vi "3.vi"() -> ()   [LabVIEW 2019]
uses:
  <vilib>/imath/engines/lvmath/Plug In/_Char/NIMS_CH_character datatype.ctl
  <vilib>/imath/engines/lvmath/Plug In/_Char/NIMS_CH_Character RV to String.vi
  <vilib>/imath/engines/lvmath2/RunTimeEngine/BuiltInFunctions/random/NIMS_random.vi
  <vilib>/imathl/engines/lvmath/Functions/Error Handling/Create Error.vi
  <vilib>/imath/engines/lvmath2/RunTimeEngine/BuiltInFunctions/fir_win/NIMS_fir_win(I32,V,Str,V,Str).vi
  <vilib>/imath/engines/lvmath2/RunTimeEngine/ErrorHandling/NIMS_Create Error From Enums.vi
  <vilib>/imath/engines/lvmath2/RunTimeEngine/BuiltInFunctions/fft/NIMS_fft(GV).vi
  <instcachedir>/0/NIMS_fft(GV)_4C6467FC22F84E4BA42517A07EF978B0.lvgen/NIMS_fft(GV)_4C6467FC22F84E4BA42517A07EF978B0_000.vi
  <vilib>/imath/engines/lvmath2/RunTimeEngine/ErrorHandling/NIMS_Error From Error Code.vi
  <vilib>/imath/engines/lvmath2/RunTimeEngine/RangeToken/NIMS_Range.vi
  <instcachedir>/0/NIMS_Range_FADF6ADDA3E145BB934C8BD4C7DAAB97.lvgen/NIMS_Range_FADF6ADDA3E145BB934C8BD4C7DAAB97_000.vi
  <vilib>/imath/engines/lvmath2/RunTimeSupport/NIMS_Error if Not Equal.vi
  <instcachedir>/0/NIMS_Error if Not Equal_D50A0F08CBFC40E0B64682CCD852CBC7.lvgen/NIMS_Error if Not Equal_D50A0F08CBFC40E0B64682CCD852CBC7_001.vi
  <vilib>/imath/engines/lvmath2/RunTimeEngine/IndexRead/NIMS V(V).vi
  <instcachedir>/0/NIMS V(V)_298D9CB7BFEB42B8BC8D9C3C28AE8C70.lvgen/NIMS V(V)_298D9CB7BFEB42B8BC8D9C3C28AE8C70_001.vi
  <vilib>/imath/engines/lvmath2/RunTimeEngine/BuiltInFunctions/abs/NIMS_abs(signed).vi
  <instcachedir>/0/NIMS_abs(signed)_C4FCB8E6058B49B797C7C8D53CA5F6EC.lvgen/NIMS_abs(signed)_C4FCB8E6058B49B797C7C8D53CA5F6EC_006.vi
  <vilib>/imath/engines/lvmath2/RunTimeEngine/BuiltInFunctions/crosscorr/NIMS_crosscorr(GM,Str).vi
  <instcachedir>/0/NIMS_crosscorr(GM,Str)_7E3A3CE9917B451394D0C3CD4C3D6955.lvgen/NIMS_crosscorr(GM,Str)_7E3A3CE9917B451394D0C3CD4C3D6955_000.vi
  <vilib>/imath/engines/lvmath2/RunTimeEngine/BuiltInFunctions/fft/NIMS_fft(GM).vi
  <instcachedir>/0/NIMS_fft(GM)_17D9014FFEBE444196AC5CE36A7D9342.lvgen/NIMS_fft(GM)_17D9014FFEBE444196AC5CE36A7D9342_000.vi
  <vilib>/imath/engines/lvmath2/RunTimeEngine/ArithmeticOperatorToken/NIMS_ArithmeticOperator_power(S).vi
  <instcachedir>/0/NIMS_ArithmeticOperator_power(S)_F1497A2DE3CE4E82B2C3646D59904248.lvgen/NIMS_ArithmeticOperator_power(S)_F1497A2DE3CE4E82B2C3646D59904248_012.vi
  <vilib>/imath/engines/lvmath2/RunTimeEngine/ArithmeticOperatorToken/NIMS_ArithmeticOperator_times.vi
  <instcachedir>/0/NIMS_ArithmeticOperator_times_B08792E9E3A74C8190DF4DEBB44E818C.lvgen/NIMS_ArithmeticOperator_times_B08792E9E3A74C8190DF4DEBB44E818C_007.vi
  <vilib>/imath/engines/lvmath2/RunTimeEngine/BuiltInFunctions/ifft/NIMS_ifft(CM).vi
  <vilib>/imath/engines/lvmath2/RunTimeEngine/BuiltInFunctions/fftshift/NIMS_fftshift(GM).vi
  <vilib>/imath/engines/lvmath2/RunTimeEngine/IndexRead/NIMS M(V).vi
  <instcachedir>/0/NIMS M(V)_948FAC22C1C943948B75DA6190348614.lvgen/NIMS M(V)_948FAC22C1C943948B75DA6190348614_005.vi
  <instcachedir>/0/NIMS_abs(signed)_C4FCB8E6058B49B797C7C8D53CA5F6EC.lvgen/NIMS_abs(signed)_C4FCB8E6058B49B797C7C8D53CA5F6EC_005.vi
  <instcachedir>/0/NIMS V(V)_298D9CB7BFEB42B8BC8D9C3C28AE8C70.lvgen/NIMS V(V)_298D9CB7BFEB42B8BC8D9C3C28AE8C70_000.vi
  <instcachedir>/0/NIMS_abs(signed)_C4FCB8E6058B49B797C7C8D53CA5F6EC.lvgen/NIMS_abs(signed)_C4FCB8E6058B49B797C7C8D53CA5F6EC_001.vi
  <vilib>/imath/engines/lvmath2/RunTimeEngine/NodeEndStatement/NIMS_NodeEndStatement_Get Vector.vi
  <instcachedir>/0/NIMS_NodeEndStatement_Get Vector_92F29E6578CC4FEABDAC0B727A70E862.lvgen/NIMS_NodeEndStatement_Get Vector_92F29E6578CC4FEABDAC0B727A70E862_001.vi
  <vilib>/imath/engines/lvmath/Functions/Error Handling/MergeErrorsWrapper.vi
  <vilib>/imath/engines/lvmath2/RunTimeEngine/NodeEndStatement/NIMS_NodeEndStatement_Output.vi
  <instcachedir>/0/NIMS_NodeEndStatement_Output_53EC0D466D134D7ABD903AC30B43404B.lvgen/NIMS_NodeEndStatement_Output_53EC0D466D134D7ABD903AC30B43404B_005.vi
  <instcachedir>/0/NIMS_NodeEndStatement_Output_53EC0D466D134D7ABD903AC30B43404B.lvgen/NIMS_NodeEndStatement_Output_53EC0D466D134D7ABD903AC30B43404B_002.vi
  <vilib>/imath/engines/lvmath2/RunTimeEngine/ErrorHandling/NIMS_Finalize Error.vi
panel:
  out "系统功率传输函数":cluster{"w":dbl[], "HW2_show":dbl[]}(graph)
  out "自相关函数":dbl[][](graph)
  out "输出信号自相关函数":dbl[][](graph)
  out "冲激响应函数":dbl[](graph)
  out "白噪声时域波形":dbl[](graph)
  out "输出信号功率谱密度":cluster{"w":dbl[], "Syy_show":dbl[]}(graph)
  out "传递函数":cluster{"w":dbl[], "HW_show":dbl[]}(graph)
  out "白噪声功率谱密度":cluster{"w":dbl[], "Sxx_show":dbl[]}(graph)
  in  "点数":dbl=500.0
  in  "上限频率":dbl=0.4
  in  "下限频率":dbl=0.3
  in  "滤波器阶数":dbl=101.0
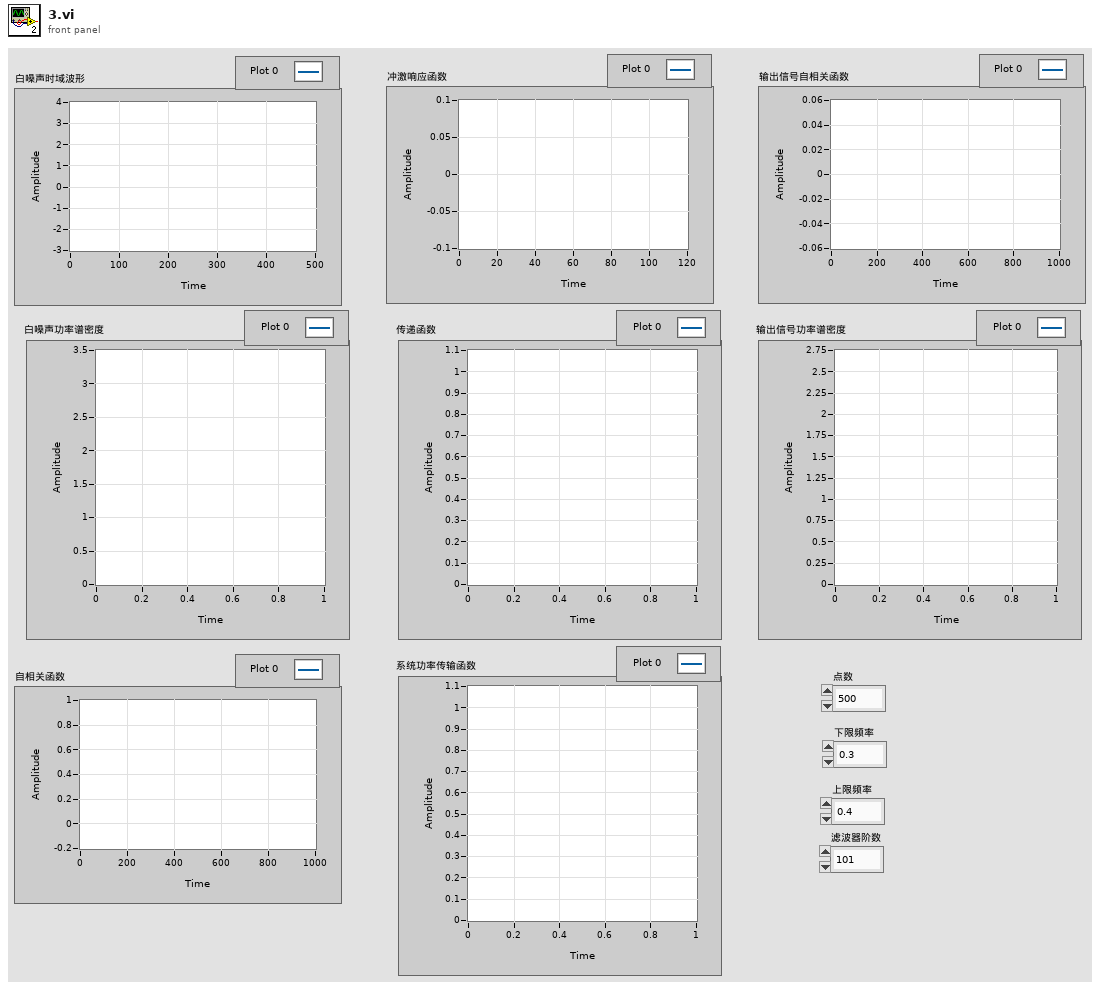
[diagram p1: front panel]
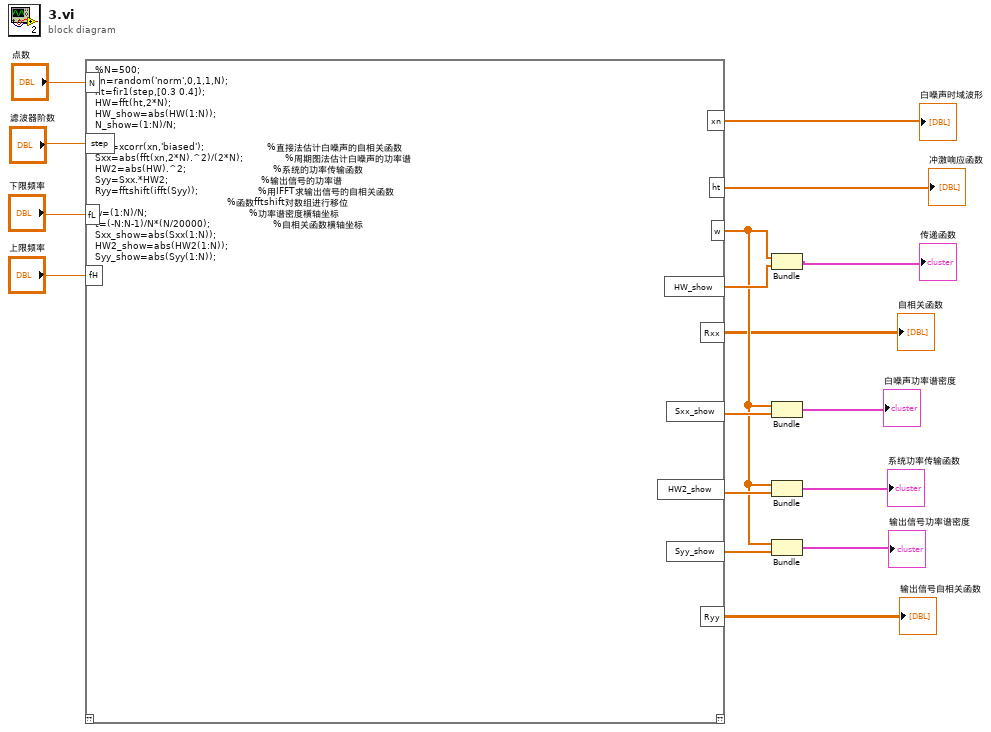
[diagram p0: block diagram]
diagram:
  n1 = mathscript code="%N=500;\nxn=random('norm',0,1,1,N);\nht=fir1(step,[0.3 0.4]);\nHW=fft(ht,2*N);\nHW_show=abs(HW(1:N));\nN_show=(1:N)/N;\n\nRxx=xcorr(xn,'biased');                     %直接法估计白噪声的自相关函数\nSxx=abs(fft(xn,2*N).^2)/(2*N);              %周期图法估计白噪声的功率谱\nHW2=abs(HW).^2;                             %系统的功率传输函数\nSyy=Sxx.*HW2;                               %输出信号的功率谱\nRyy=fftshift(ifft(Syy));                    %用IFFT求输出信号的自相关函数\n                                            %函数fftshift对数组进行移位\nw=(1:N)/N;                                  %功率谱密度横轴坐标\nt=(-N:N-1)/N*(N/20000);                     %自相关函数横轴坐标\nSxx_show=abs(Sxx(1:N));\nHW2_show=abs(HW2(1:N));\nSyy_show=abs(Syy(1:N));"("step"="滤波器阶数", "fL"="下限频率", "fH"="上限频率", "N"="点数") -> ("xn"=→"白噪声时域波形":dbl[], "ht"=→"冲激响应函数":dbl[], "HW_show"=w13:dbl[], "Rxx"=→"自相关函数":dbl[][], "Sxx_show"=w12:dbl[], "HW2_show"=w11:dbl[], "Syy_show"=w10:dbl[], "Ryy"=→"输出信号自相关函数":dbl[][], "w"=w9:dbl[])  [unwired: 1 in, 1 out]
  n2 = Bundle("w"=w9, "HW_show"=w13) -> (→"传递函数":cluster{"w":dbl[], "HW_show":dbl[]})  [unwired: 1 in]
  n3 = Bundle("w"=w9, "Sxx_show"=w12) -> (→"白噪声功率谱密度":cluster{"w":dbl[], "Sxx_show":dbl[]})  [unwired: 1 in]
  n4 = Bundle("w"=w9, "HW2_show"=w11) -> (→"系统功率传输函数":cluster{"w":dbl[], "HW2_show":dbl[]})  [unwired: 1 in]
  n5 = Bundle("w"=w9, "Syy_show"=w10) -> (→"输出信号功率谱密度":cluster{"w":dbl[], "Syy_show":dbl[]})  [unwired: 1 in]
